vi "Configure.vi"(8 "error in (no error)":errorcluster) -> (0 "error out":errorcluster, 1 "valid configuration":bool, 3 "config":T1)   [LabVIEW 2017, in "BurstMode.lvlib"]
uses:
  <vilib>/addons/InsightCM/Devices/Shared/Cms/CmsBurstMode/BurstMode.lvlib
  <vilib>/addons/InsightCM/Devices/Shared/Cms/CmsBurstMode/controls/config.ctl
  <vilib>/addons/InsightCM/Utilities/GlobalConfiguration/GlobalConfiguration.lvlib
  <vilib>/addons/InsightCM/Devices/Shared/Cms/CmsAcquisition/CmsAcquisition.lvlib
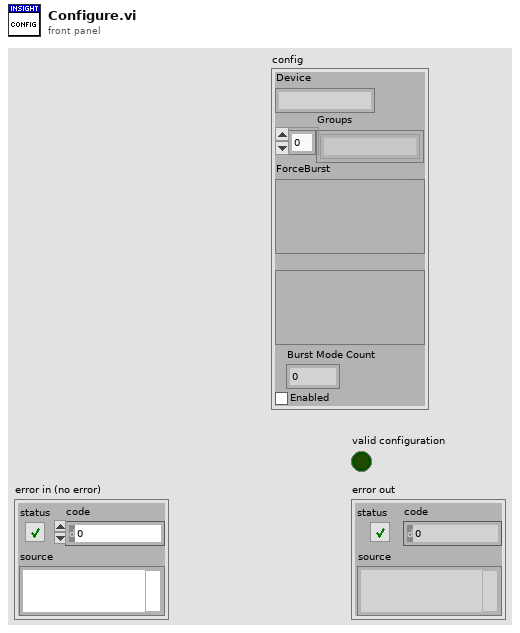
[diagram p1: front panel]
types:
  T1 = typedef "BurstMode.lvlib/config.ctl" = cluster{"Device":string, "Groups":string[], "ForceBurst":variant, "TriggerBurst":variant, "Burst Mode Count":i32, "Enabled":bool}
  T2 = typedef "R2_Device.ctl" = cluster{"Id":string, "Name":string, "DeviceType":string, "HardwareName":string, "IpAddress":string, "HardwareInfo":T3[], "ApplicationType":string, "ApplicationVersion":string, "EquipmentIds":string[], "ConfigurationVersion":string, "State":T4, "Properties":T3[], "DataGroups":T5[], "BurstModeTrigger":T9}
  T3 = typedef "KeyValuePair.ctl" = cluster{"Key":string, "Value":string}
  T4 = typedef "DeviceState.ctl" = cluster{"Disabled":bool}
  T5 = typedef "R2_DataGroup.ctl" = cluster{"Name":string, "OperatingStates":T6[], "Properties":T3[], "EquipmentIds":string[], "AssetNodeId":string}
  T6 = typedef "OperatingState.ctl" = cluster{"Name":string, "Properties":T3[], "Triggers":T7[]}
  T7 = typedef "Trigger.ctl" = cluster{"Type":string, "Expression":string, "Conditions":T8[]}
  T8 = typedef "Condition.ctl" = cluster{"Source":string, "Type":string, "Operator":string, "CompareTo":string, "DwellSeconds":dbl}
  T9 = typedef "BurstModeTrigger.ctl" = cluster{"Trigger":T7, "SampleRate":string, "AcquisitionLength":string}
  T10 = typedef "MetricDefinitionInstance.ctl" = cluster{"Id":string, "MetricType":string, "Name":string, "Properties":T3[], "HighRate":bool}
  T11 = typedef "SectionKeyValues.ctl" = cluster{"Section":string, "KeyValues":T3[]}
  T12 = typedef "AssetNode.ctl" = cluster{"Id":string, "Type":string, "Name":string, "ParentIds":string[], "State":T13, "MeasType":string, "Properties":T3[], "OperatingStates":T6[], "Metrics":T14[], "TrendAlarmRules":T15[], "References":T18[]}
  T13 = typedef "AssetState.ctl" = cluster{"Disabled":bool}
  T14 = typedef "Metric.ctl" = cluster{"Id":string, "Name":string, "Unit":string, "Properties":T3[], "MetricDefinitionInstanceId":string}
  T15 = typedef "TrendAlarmRule.ctl" = cluster{"Id":string, "AssetNodeId":string, "TrendId":string, "Disabled":bool, "OperatingState":string, "Operator":string, "Hysteresis":dbl, "OnDelaySeconds":dbl, "OffDelaySeconds":dbl, "Levels":T16[], "Properties":T3[]}
  T16 = typedef "TrendAlarmLevel.ctl" = cluster{"Severity":i32, "CompareTo":dbl, "Actions":T17[]}
  T17 = typedef "AlarmAction.ctl" = cluster{"Type":string, "Props":T3[]}
  T18 = typedef "AssetNodeReference.ctl" = cluster{"NodeId":string, "Name":string}
  T19 = typedef "R2_Channel.ctl" = cluster{"Id":string, "DeviceId":string, "Name":string, "ChannelType":string, "HardwareKey":string, "HardwareChannel":string, "DataGroup":string, "Keywords":string[], "EquipmentIds":string[], "Properties":T3[], "Metrics":T14[], "AssetNodeId":string, "MeasType":string, "AssetName":string}
  T20 = typedef "BurstMode.lvlib/device.ctl" = cluster{"Name":string, "Properties":T3[], "BurstExpression":string, "BurstConditions":T21[]}
  T21 = typedef "Trigger.lvlib/TriggerCondition.ctl" = cluster{"Condition":T8, "LatchValue":string, "LatchTime":timestamp}
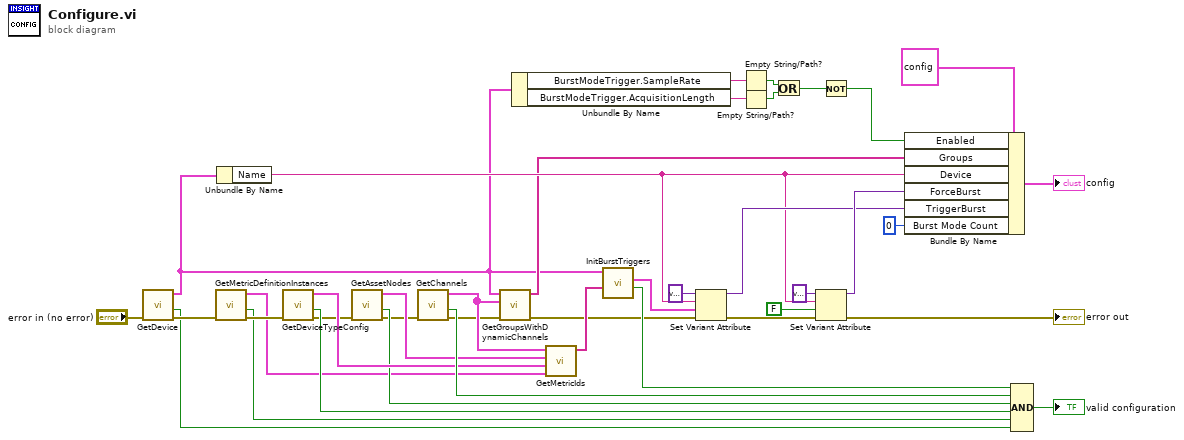
[diagram p0: block diagram]
diagram:
  n1 = call <vilib>:"GetDevice.vi"("error in (no error)"="error in (no error)") -> ("error out"=w28:errorcluster, "found"=w25:bool, "device configuration"=w7:T2)  [unwired: 8 in]
  n2 = call <vilib>:"GetMetricDefinitionInstances.vi"("error in (no error)"=w28) -> ("error out"=w27:errorcluster, "found"=w24:bool, "metrics"=w26:T10[])  [unwired: 8 in]
  n3 = Unbundle By Name(w7) -> ("Name"=w14:string)
  n4 = call <vilib>:"GetDeviceTypeConfig.vi"("error in (no error)"=w27) -> ("error out"=w30:errorcluster, "found"=w33:bool, "key values"=w34:T11[])  [unwired: 8 in]
  n5 = call <vilib>:"GetAssetNodes.vi"("error in (no error)"=w30) -> ("error out"=w29:errorcluster, "found"=w32:bool, "AssetNodes"=w31:T12[])  [unwired: 8 in]
  n6 = call <vilib>:"GetChannels.vi"("error in (no error)"=w29) -> ("error out"=w9:errorcluster, "found"=w35:bool, "channels"=w11:T19[])  [unwired: 8 in]
  n7 = call <vilib>:"GetGroupsWithDynamicChannels.vi"("error in (no error)"=w9, "channels"=w11, "device configuration"=w7) -> ("error out"=w8:errorcluster, "groups with dynamic channels"=w10:string[])  [unwired: 7 in]
  n8 = Unbundle By Name(w7) -> ("BurstModeTrigger.SampleRate"=w6:string, "BurstModeTrigger.AcquisitionLength"=w5:string)
  n9 = call <vilib>:"GetMetricIds.vi"("metrics"=w26, "device type config"=w34, "AssetNodes"=w31, "channels"=w11) -> ("metric ids"=w19:string[])  [unwired: 7 in]
  n10 = call <vilib>:"InitBurstTriggers.vi"("metric ids"=w19, "device configuration"=w7) -> ("valid config"=w18:bool, "device"=w17:T20)  [unwired: 8 in]
  n11 = Set Variant Attribute(Variant=variant ("Status"), name=w14, value=w17, error in=w8) -> (Variant out=w37:variant, error out=w21:errorcluster)  [unwired: 1 out]
  n12 = Empty String/Path?(string/path=w6) -> (empty?=w4:bool)
  n13 = Empty String/Path?(string/path=w5) -> (empty?=w3:bool)
  n14 = Or(x=w4, y=w3) -> (x .or. y?=w2:bool)
  n15 = Set Variant Attribute(Variant=variant ("Status"), name=w14, value=FALSE ("ForceTrigger"), error in=w21) -> (Variant out=w38:variant, error out=→"error out":errorcluster)  [unwired: 1 out]
  n16 = Not(x=w2) -> (.not. x?=w1:bool)
  n17 = Bundle By Name(cluster=T1 {"Device"="", "Groups"=[], "ForceBurst"=variant, "TriggerBurst"=variant, "Burst Mode Count"=0, "Enabled"=FALSE} ("config"), "Enabled"=w1, "Groups"=w10, "Device"=w14, "ForceBurst"=w38, "TriggerBurst"=w37, "Burst Mode Count"=0) -> (→"config":T1)
  n18 = Compound Arithmetic op=AND(w18, w35, w32, w33, w24, w25) -> (→"valid configuration":bool)
